vi "Get Control Panel VI Path.vi"(8 "error in (no error)":errorcluster, 11 "IPS120 in":refnum<class "IPS120.lvclass">) -> (0 "error out":errorcluster, 2 "Front Panel VI path":path, 3 "IPS120 out":refnum<class "IPS120.lvclass">)   [LabVIEW 2015, in "IPS120.lvclass"]
uses:
  IPS120.lvclass
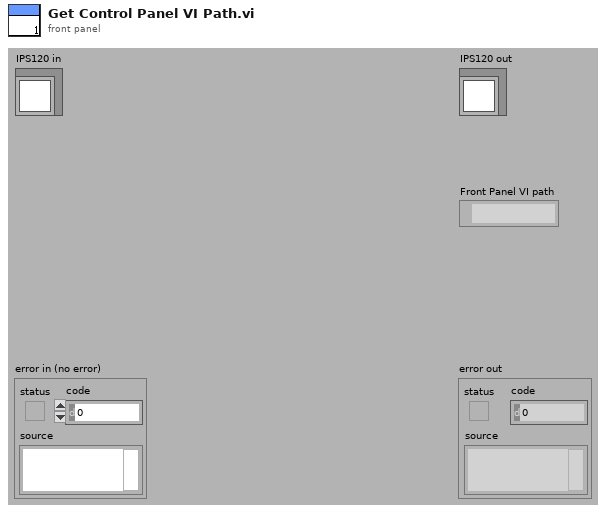
[diagram p1: front panel]
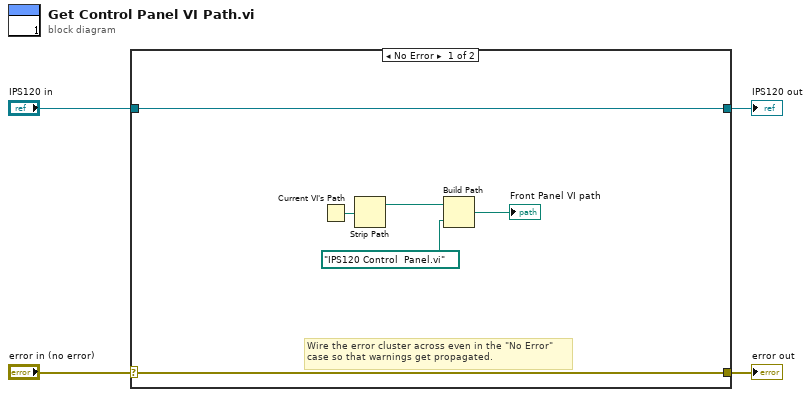
[diagram p0: block diagram]
diagram:
  n1 = case shown="No Error" "error in (no error)" {
    selector: "error in (no error)" -> [w9 w12]
    tunnel: [w9 w12] -> w3
    tunnel: [w10 w11] -> w1
    tunnel: "IPS120 in" -> [w10 w11]
    frame No Error {
      # "Wire the error cluster across even in the \"No Error\"\ncase so that warnings get propagated."
      n2 = Current VI's Path() -> (path=w6:path)
      n3 = Strip Path(path=w6) -> (stripped path=w7:path)  [unwired: 1 out]
      n4 = Build Path(base path=w7, name or relative path=path "IPS120 Control  Panel.vi") -> (appended path=→"Front Panel VI path":path)
    }
    frame Error {
    }
  }
  "error out" <- w3
  "IPS120 out" <- w1
